vi "find zero crossings detector backup.vi"(0 "display queues":T1, 5 "slope":bool=TRUE, 7 "hysteresis":dbl=0.05 format="%#_13g", 11 "error in (no error)":errorcluster) -> (2 "crossing stats":T3, 3 "period":dbl, 4 "recent crossing":dbl, 6 "prev crossing":dbl, 8 "crossing-2":dbl, 10 "new crossing":bool, 14 "number of crossings":i32, 15 "error out":errorcluster)   [LabVIEW 2017]
uses:
  typedefs/queue cluster.ctl
  typedefs/reading queue.ctl
  typedefs/reading.ctl
  typedefs/readingType.ctl
panel:
  in  "disk queues":T1
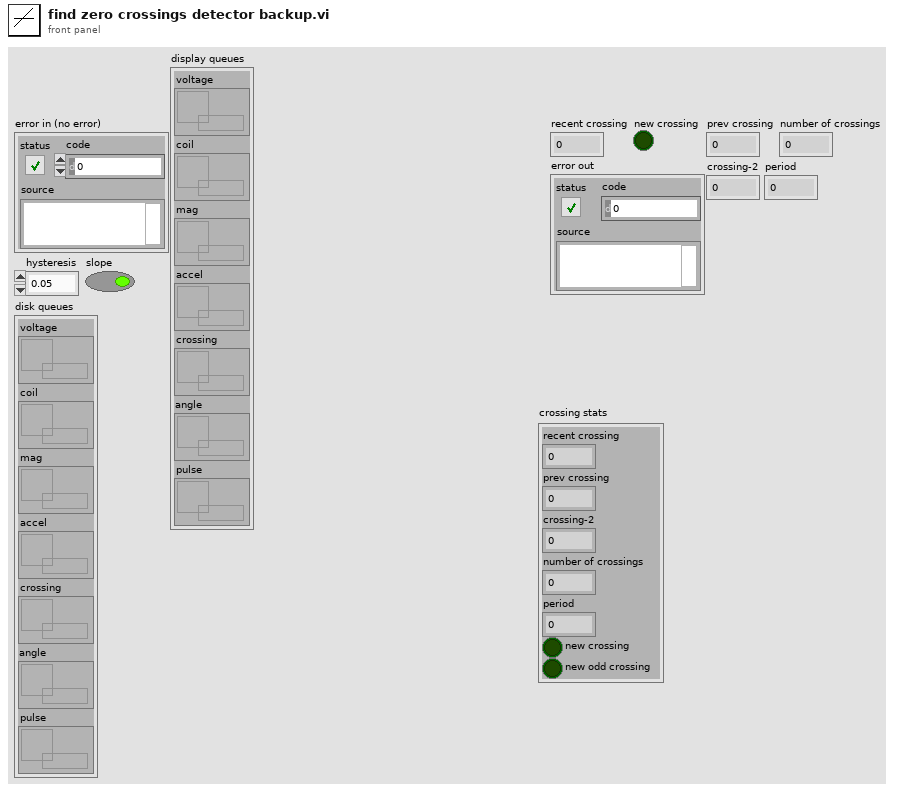
[diagram p1: front panel]
types:
  T1 = typedef "queue cluster.ctl" = cluster{"voltage":T2, "coil":T2, "mag":T2, "accel":T2, "crossing":T2, "angle":T2, "pulse":T2}
  T2 = typedef "reading queue.ctl" = refnum<queue>
  T3 = cluster{"recent crossing":dbl, "prev crossing":dbl, "crossing-2":dbl, "number of crossings":i32, "period":dbl, "new crossing":bool, "new odd crossing":bool}
  T4 = typedef "reading.ctl" = cluster{"reading type":T5, "time":fxp<+,48,48>, "x":sgl, "y":sgl, "z":sgl, "XSUM":u8}
  T5 = typedef "readingType.ctl" = enum8{"SYNC", "DETVAL", "COILI", "MAGVEC", "ACCVEC", "CROSSING"}
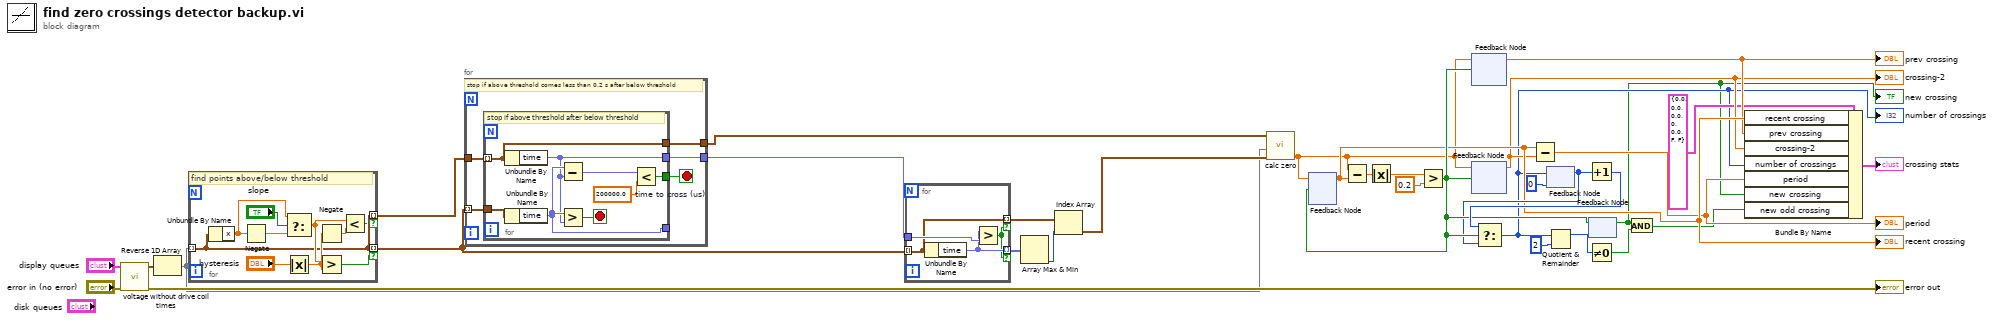
[diagram p0: block diagram]
diagram:
  n1 = call "voltage without drive coil times.vi"("error in (no error)"="error in (no error)", "display queues"="display queues") -> ("error out"=→"error out":errorcluster, "voltage_no_coil"=w22:T4[])  [unwired: 7 in, 1 out]
  n2 = Reverse 1D Array(array=w22) -> (reversed array=w1:T4[])
  n3 = for {
    tunnel: w1 -> [w35] mode=indexing
    tunnel: [w35] -> w29 mode=indexing if=w39
    tunnel: [w35] -> w33 mode=indexing if=w34
    # "find points above/below threshold"
    n4 = Unbundle By Name(w35) -> ("x"=w42:sgl)
    n5 = Negate(x=w42) -> (-x=w41:sgl)
    n6 = Select(t=w42, s="slope", f=w41) -> (s? t:f=w36:sgl)
    n7 = Absolute Value(x="hysteresis") -> (abs(x)=w38:dbl)
    n8 = Negate(x=w38) -> (-x=w37:dbl)
    n9 = Greater?(x=w36, y=w38) -> (0:w39:bool)
    n10 = Less?(x=w36, y=w37) -> (x < y?=w34:bool)
  }
  n11 = for {
    tunnel: w29 -> [w48] mode=indexing
    tunnel: w33 -> [w47]
    tunnel: [w45] -> w28
    tunnel: [w44] -> w24
    stop <- w46 stop-if-true
    # "stop if above threshold comes less than 0.2 s after below threshold"
    n12 = for {
      tunnel: w48 -> [w56]
      tunnel: w47 -> [w49] mode=indexing
      tunnel: [w52] -> w46
      tunnel: [w51] -> _
      tunnel: [w50] -> w45
      tunnel: [w49] -> w44
      stop <- w55 stop-if-true
      w53 = 200000.0  # time to cross (us)
      # "stop if above threshold after below threshold"
      n13 = Unbundle By Name(w49) -> ("time"=w50:fxp<+,48,48>)
      n14 = Unbundle By Name(w56) -> ("time"=w51:fxp<+,48,48>)
      n15 = Subtract(x=w51, y=w50) -> (x-y=w54:fxp<+/-,49,49>)
      n16 = Greater?(x=w51, y=w50) -> (0:w55:bool)
      n17 = Less?(x=w54, y=w53) -> (x < y?=w52:bool)
    }
  }
  n18 = for {
    tunnel: w29 -> [w59] mode=indexing
    tunnel: w28 -> [w60]
    tunnel: [w59] -> w26 mode=indexing if=w57
    tunnel: [w58] -> w27 mode=indexing if=w57
    n19 = Unbundle By Name(w59) -> ("time"=w58:fxp<+,48,48>)
    n20 = Greater?(x=w58, y=w60) -> (0:w57:bool)
  }
  n21 = Array Max & Min(array=w27) -> (min index (indices)=w25:i32)  [unwired: 3 out]
  n22 = Index Array(array=w26, index=w25) -> (element=w23:T4)
  n23 = call "calc zero.vi"("voltage"=w1, "stop reading"=w23, "start reading"=w24) -> ("tcross (s)"=w2:dbl)  [unwired: 8 in]
  n24 = feedback #1() -> (w15:dbl)  [unwired: 1 in]
  "recent crossing" <- w15
  n25 = Subtract(x=w2, y=w15) -> (x-y=w32:dbl)
  n26 = Absolute Value(x=w32) -> (abs(x)=w31:dbl)
  n27 = Greater?(x=w31, y=0.2) -> (0:w17:bool)
  n28 = feedback-in #1(w2, w17) -> ()
  n29 = feedback-in #2(w2, w17) -> ()
  n30 = feedback #2() -> (w14:dbl)  [unwired: 1 in]
  "prev crossing" <- w14
  n31 = feedback #3() -> (w13:dbl)  [unwired: 1 in]
  "crossing-2" <- w13
  n32 = feedback-in #3(w2, w17) -> ()
  n33 = Subtract(x=w15, y=w13) -> (x-y=w12:dbl)
  "period" <- w12
  n34 = feedback #4(0) -> (w16:i32)
  n35 = Increment(x=w16) -> (x+1=w19:i32)
  n36 = Select(t=w19, s=w17, f=w16) -> (s? t:f=w9:i32)
  "number of crossings" <- w9
  n37 = feedback-in #4(w9) -> ()
  n38 = Quotient & Remainder(x=w9, y=2) -> (x-y*floor(x/y)=w7:i32)  [unwired: 1 out]
  n39 = Not Equal To 0?(x=w7) -> (x != 0?=w6:bool)
  n40 = feedback-in #5(w17) -> ()
  n41 = feedback #5() -> (w5:bool)  [unwired: 1 in]
  "new crossing" <- w5
  n42 = And(x=w5, y=w6) -> (x .and. y?=w4:bool)
  n43 = Bundle By Name(cluster=T3 {"recent crossing"=0.0, "prev crossing"=0.0, "crossing-2"=0.0, "number of crossings"=0, "period"=0.0, "new crossing"=FALSE, "new odd crossing"=FALSE} ("crossing stats"), "recent crossing"=w15, "prev crossing"=w14, "crossing-2"=w13, "number of crossings"=w9, "period"=w12, "new crossing"=w5, "new odd crossing"=w4) -> (→"crossing stats":T3)
